vi "Array Comparision.vi"() -> ()   [LabVIEW 2015]
panel:
  in  "stop":bool
  out "Array 2":bool[](array[boolean])
  in  "Array":dbl[](array[numeric])
  # "Array Comparision"
  # "Pardeep Kumar"
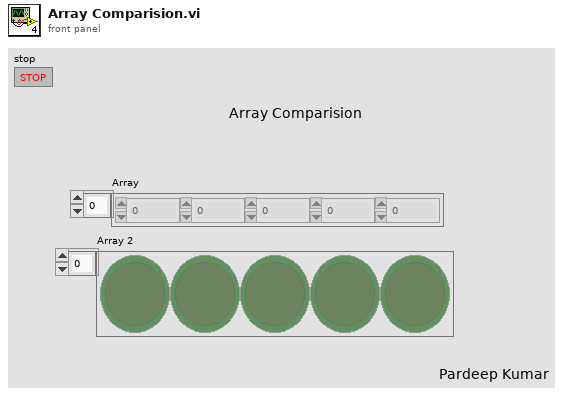
[diagram p1: front panel]
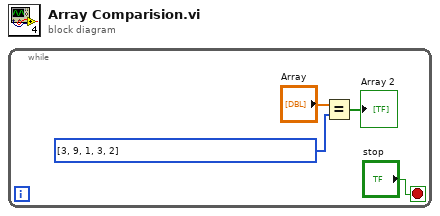
[diagram p0: block diagram]
diagram:
  n1 = while {
    stop <- "stop" stop-if-true
    n2 = Equal?(x="Array", y=i32[] [3, 9, 1, 3, 2]) -> (x = y?=→"Array 2":bool[])
  }
